vi "Find Instruments.vi"(8 "error in (no error)":errorcluster, 11 "Instrument Detection in":refnum<class "Instrument Detection.lvclass">) -> (0 "error out":errorcluster, 3 "Instrument Detection out":refnum<class "Instrument Detection.lvclass">)   [LabVIEW 2020, in "Instrument Detection.lvlib" / "Instrument Detection.lvclass"]
doc: "Incomplete VI!"
uses:
  Instrument Detection.lvclass
  Controls/Ctl_IDStringType.ctl
  35f783f7-1bce-4f81-8e86-95c97776ac01.vi
  Instrument Detection.lvlib
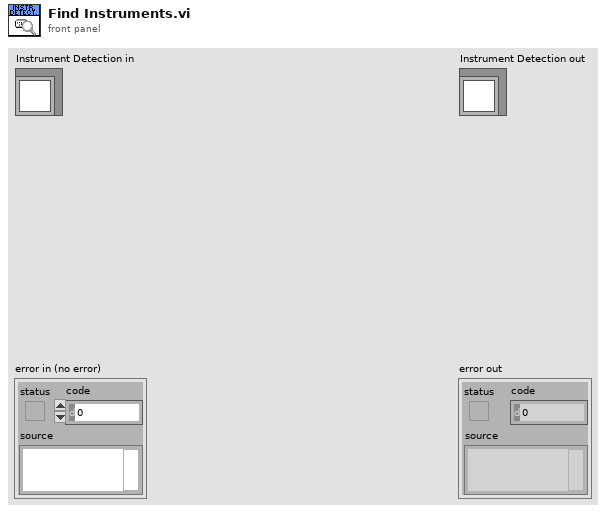
[diagram p1: front panel]
types:
  T1 = typedef "Instrument Detection.lvlib/Ctl_IDStringType.ctl" = enum16{"Serial Number", "Product Name", "Vendor Name", "Description"}
  T2 = typedef "Instrument Detection.lvlib/Ctl_NI MAX Device Info.ctl" = cluster{"Alias":string, "Product Name":string, "Vendor Name":string, "Serial Number":string, "Connection":T3, "Description":string, "ID":string, "Owner":string}
  T3 = typedef "HDH.Actor Framework.Core.Instrument Driver.lvlibp/Instrument Driver.lvclass/Ctl_ConnectionType.ctl" = enum16{"BuiltIn/System", "PXI/PCI", "USB", "GPIB", "VXI", "Serial", "TCP/IP", "cRIO", "SCXI", "cDAQ", "SwitchBlock", "SCC", "FireWire", "Accessory", "CAN", "SwitchBlock Device"}
  T4 = typedef "Instrument Detection.lvlib/Ctl_InstrumentID.ctl" = cluster{"Driver Name":string, "Instrument ID":u32}
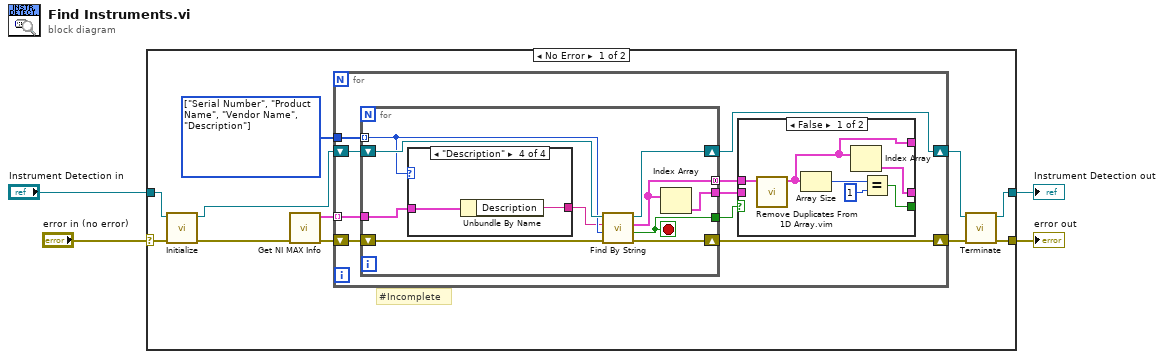
[diagram p0: block diagram]
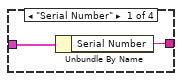
[diagram p3: hidden frame]
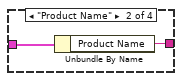
[diagram p4: hidden frame]
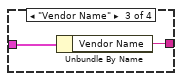
[diagram p5: hidden frame]
diagram:
  n1 = case shown="No Error" "error in (no error)" {
    selector: "error in (no error)" -> [w15 w52]
    tunnel: [w5 w52] -> w3
    tunnel: [w7 w51] -> w1
    tunnel: "Instrument Detection in" -> [w14 w51]
    frame No Error {
      w12 = T1[] [enum."Serial Number", enum."Product Name", enum."Vendor Name", enum."Description"] items=["Serial Number", "Product Name", "Vendor Name", "Description"] ("Array")
      # "#Incomplete"
      n2 = call-dynamic "Initialize.vi"("error in (no error)"=w15, "Instrument Detection in"=w14) -> ("error out"=w11:errorcluster, "Instrument Detection out"=w13:refnum<class "Instrument Detection.lvclass">)  [unwired: 8 in]
      n3 = call "Get NI MAX Info.vi"("error in (no error)"=w11) -> ("error out"=w9:errorcluster, "Device Info"=w10:T2[])  [unwired: 9 in]
      n4 = for {
        tunnel: w12 -> [w23]
        tunnel: w10 -> [w22] mode=indexing
        shift-right: [w19] -> w6
        shift-left: w9 -> [w21]
        shift-right: [w20] -> w8
        shift-left: w13 -> [w24]
        n5 = for {
          tunnel: w23 -> [w41] mode=indexing
          tunnel: w22 -> [w40]
          shift-right: [w37] -> w19
          shift-left: w21 -> [w38]
          shift-right: [w36] -> w20
          shift-left: w24 -> [w42]
          tunnel: [w35] -> w18
          tunnel: [w34] -> w16 mode=concatenating
          tunnel: [w33] -> w17
          stop <- w35 stop-if-true
          n6 = case shown="\"Description\"" w41 {
            tunnel: w40 -> [w44 w46 w48 w50]
            tunnel: [w43 w45 w47 w49] -> w39
            frame "Serial Number" {
              n7 = Unbundle By Name(w44) -> ("Serial Number"=w43:string)
            }
            frame "Product Name" {
              n8 = Unbundle By Name(w46) -> ("Product Name"=w45:string)
            }
            frame "Vendor Name" {
              n9 = Unbundle By Name(w48) -> ("Vendor Name"=w47:string)
            }
            frame "Description" {
              n10 = Unbundle By Name(w50) -> ("Description"=w49:string)
            }
          }
          n11 = call-dynamic "Find By String.vi"("error in (no error)"=w38, "ID String Type"=w41, "Identification String"=w39, "Instrument Detection in"=w42) -> ("error out"=w37:errorcluster, "Uniquely Identified?"=w35:bool, "Possible Instruments"=w34:T4[], "Instrument Detection out"=w36:refnum<class "Instrument Detection.lvclass">)  [unwired: 4 in]
          n12 = Index Array(array=w34) -> (element=w33:T4)  [unwired: 1 in]
        }
        n13 = case shown="False" w18 {
          selector: w18 -> [_ w31]
          tunnel: w17 -> [_ w32]
          tunnel: [w28 w32] -> _
          tunnel: w16 -> [w26 _]
          tunnel: [w27 w31] -> _
          tunnel: [w25 _] -> _
          frame False {
            n14 = call "Remove Duplicates From 1D Array.vim"("array"=w26) -> ("array with duplicates removed"=w25:T4[])  [unwired: 10 in]
            n15 = Array Size(array=w25) -> (size(s)=w30:i32)
            n16 = Index Array(array=w25) -> (element=w28:T4)  [unwired: 1 in]
            n17 = Equal?(x=w30, y=1) -> (x = y?=w27:bool)
          }
          frame True {
          }
        }
      }
      n18 = call-dynamic "Terminate.vi"("error in (no error)"=w6, "Instrument Detection in"=w8) -> ("error out"=w5:errorcluster, "Instrument Detection out"=w7:refnum<class "Instrument Detection.lvclass">)  [unwired: 8 in]
    }
    frame Error {
    }
  }
  "error out" <- w3
  "Instrument Detection out" <- w1
